vi "Encode (Single).vi"(8 "error in (no error)":errorcluster, 10 "Data":string, 11 "QR Code Encoder in":refnum<class "QR Code Encoder.lvclass">) -> (0 "error out":errorcluster, 2 "QR Code Image Data":u8[][](array[numeric]), 3 "QR Code Encoder":refnum<class "QR Code Encoder.lvclass">)   [LabVIEW 2020, in "feature_detection.lvlib" / "QR Code Encoder.lvclass"]
doc: "Encode the supplied Data into QR Code Image Data."
uses:
  QR Code Encoder.lvclass
  QR Code Encoder.lvclass/QR Code Encoder.ctl
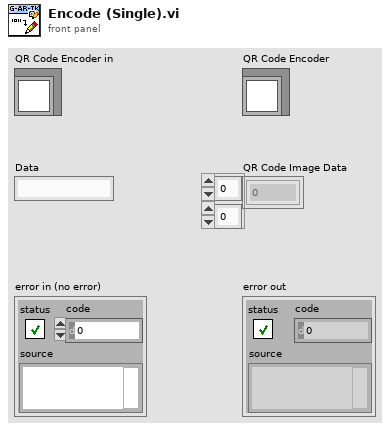
[diagram p1: front panel]
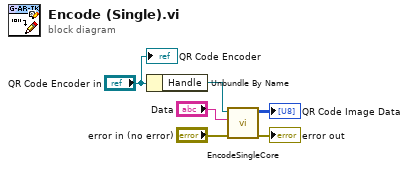
[diagram p0: block diagram]
diagram:
  n1 = Unbundle By Name("QR Code Encoder in") -> ("Handle"=w5:refnum<data-value>)
  n2 = call "EncodeSingleCore.vi"("error in (no error)"="error in (no error)", "Data"="Data", "Data Value Reference in"=w5) -> ("error out"=→"error out":errorcluster, "QR Code Image Data"=→"QR Code Image Data":u8[][])  [unwired: 7 in]
  "QR Code Encoder" <- "QR Code Encoder in"
